vi "MS Is array same.vi"(3 "Array":dbl[](array[numeric])) -> (1 "Ready":bool)   [LabVIEW 2017, in "Magnet module.lvlib"]
doc: "Compares all values of array and check if they have the same."
uses:
  Magnet module.lvlib
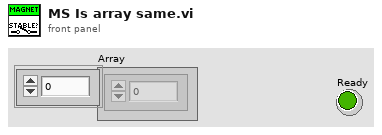
[diagram p1: front panel]
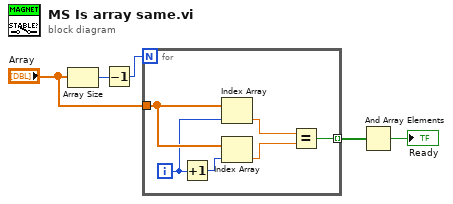
[diagram p0: block diagram]
diagram:
  n1 = Array Size(array="Array") -> (size(s)=w3:i32)
  n2 = Decrement(x=w3) -> (x-1=w4:i32)
  n3 = for {
    N: w4 -> [_]
    tunnel: "Array" -> [w11]
    tunnel: [w10] -> w5 mode=indexing
    i -> [w9]
    n4 = Increment(x=w9) -> (x+1=w8:i32)
    n5 = Index Array(array=w11, index=w9) -> (element=w7:dbl)
    n6 = Index Array(array=w11, index=w8) -> (element=w6:dbl)
    n7 = Equal?(x=w7, y=w6) -> (x = y?=w10:bool)
  }
  n8 = And Array Elements(Boolean array=w5) -> (logical AND=→"Ready":bool)
